vi "To String and From String Array Test.vi"() -> ()   [LabVIEW 2018, in "Wait on Integer Tests.lvlib"]
uses:
  Wait on Integer Tests.lvlib
  <vilib>/NI/Tag Bus/tag/Data Type.ctl
  <vilib>/NI/Tag Bus Module Framework/channel/channel classification.ctl
  Config/Wait On Integer Config.lvclass
  Config/Wait On Integer Config.lvclass/Wait On Integer Config.ctl
  Config/Write Wait On Integer Event.vi
  Config/Write Target Integer.vi
  Config/Write Timeout.vi
  Config/Read Wait On Integer Event.vi
  Config/Read Target Integer.vi
  Config/Read Timeout.vi
  <vilib>/NI/Tag Bus Module Framework/channel/TBM channel.lvclass
  <vilib>/NI/Tag Bus/tag/tag descriptor.lvclass
panel:
  out "Timeout Equal?":bool
  out "Target Integer Equal?":bool
  out "Channel Equal?":bool
  out "Pass?":bool
  out "error out":errorcluster
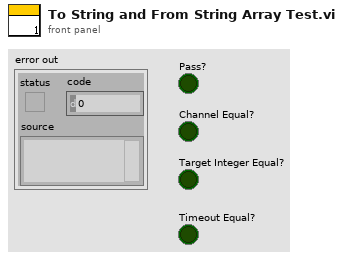
[diagram p1: front panel]
types:
  T1 = typedef "TBM channel.lvclass/channel classification.ctl" = enum16{"input data", "output data", "processing parameter", "processing result"}
  T2 = typedef "tag bus.lvlib/tag descriptor.lvclass/Data Type.ctl" = enum16{"Double", "Single", "I64", "I32", "I16", "I8", "U64", "U32", "U16", "U8", "Boolean", "String", "Array of Double", "Array of Single", "Array of I64", "Array of I32", "Array of I16", "Array of I8", "Array of U64", "Array of U32", "Array of U16", "Array of U8", "Array of Boolean", "Array of String"}
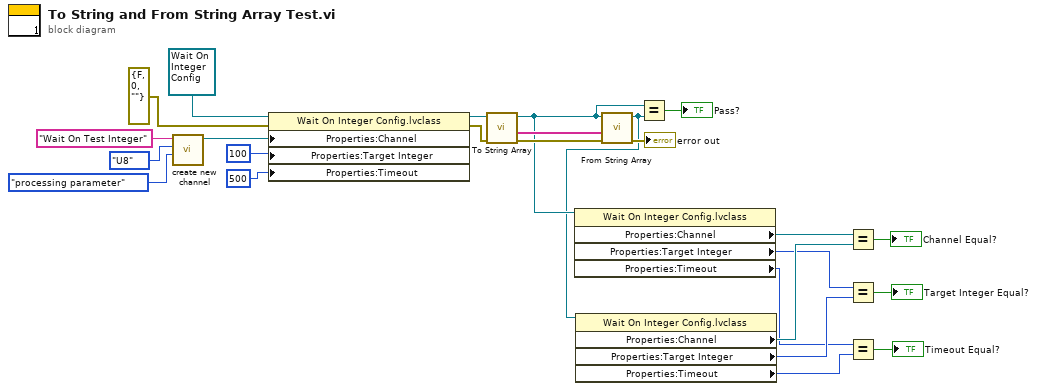
[diagram p0: block diagram]
diagram:
  n1 = call <vilib>:"create new channel.vi"("channel classification"=channel_classification."processing parameter", "data type"=Data_Type."U8", "channel name"="Wait On Test Integer") -> ("channel"=w24:refnum<class "TBM channel.lvclass">)  [unwired: 8 in]
  n2 = property class="Wait On Integer Config.lvclass"(reference=refnum<class "Wait On Integer Config.lvclass"> refnum ("Wait On Integer Step Config.lvclass"), error in=errorcluster {"status"=FALSE, "code"=0, "source"=""} ("error in (no error)"), "Properties:Channel"=w24, "Properties:Target Integer"=u32 100 ("Target Integer"), "Properties:Timeout"=500 ("Timeout")) -> (reference out=w23:refnum<class "Wait On Integer Config.lvclass">, error out=w20:errorcluster)
  n3 = call-dynamic "To String Array.vi"("error in (no error)"=w20, "Wait On Integer Step Config in"=w23) -> ("error out"=w19:errorcluster, "Step String Array"=w16:string[], "Wait On Integer Step Config out"=w11:refnum<class "Wait On Integer Config.lvclass">)  [unwired: 7 in]
  n4 = property class="Wait On Integer Config.lvclass"(reference=w11) -> ("Properties:Channel"=w9:refnum<class "TBM channel.lvclass">, "Properties:Target Integer"=w6:u32, "Properties:Timeout"=w5:i32)  [unwired: 1 in, 2 out]
  n5 = call-dynamic "From String Array.vi"("error in (no error)"=w19, "String Array"=w16, "Wait On Integer Step Config in"=w11) -> ("error out"=→"error out":errorcluster, "Wait On Integer Step Config out"=w10:refnum<class "Wait On Integer Config.lvclass">)  [unwired: 5 in, 2 out]
  n6 = property class="Wait On Integer Config.lvclass"(reference=w10) -> ("Properties:Channel"=w8:refnum<class "TBM channel.lvclass">, "Properties:Target Integer"=w7:u32, "Properties:Timeout"=w4:i32)  [unwired: 1 in, 2 out]
  n7 = Equal?(x=w11, y=w10) -> (x = y?=→"Pass?":bool)
  n8 = Equal?(x=w9, y=w8) -> (x = y?=→"Channel Equal?":bool)
  n9 = Equal?(x=w6, y=w7) -> (x = y?=→"Target Integer Equal?":bool)
  n10 = Equal?(x=w5, y=w4) -> (x = y?=→"Timeout Equal?":bool)
